vi "Send Hardware Reference.vi"(8 "error in":errorcluster, 11 "Controller in":refnum<class "Controller.lvclass">) -> (0 "error out":errorcluster, 2 "System Hardware Reference":refnum<data-value>, 3 "Controller out":refnum<class "Controller.lvclass">)   [LabVIEW 2016, in "SMI.lvlib" / "Controller.lvclass"]
uses:
  Controller.lvclass
  Controller.lvclass/Controller.ctl
  Accessor Methods/Read System Hardware Reference.vi
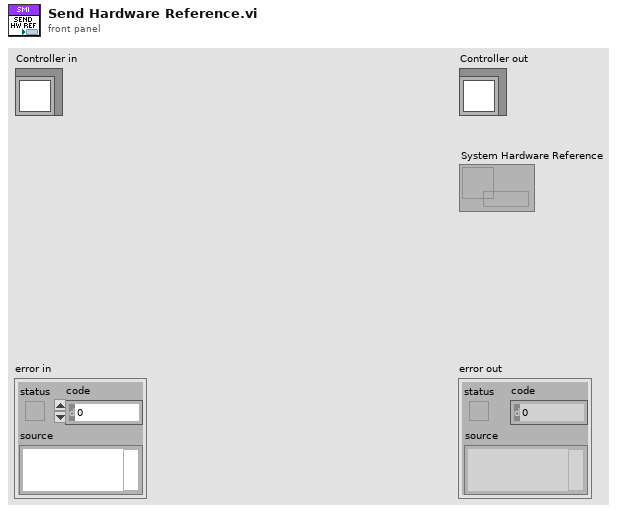
[diagram p1: front panel]
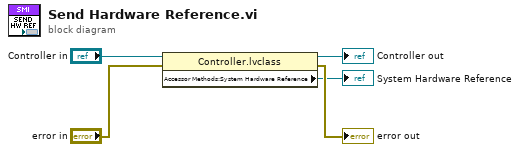
[diagram p0: block diagram]
diagram:
  n1 = property class="Controller.lvclass"(reference="Controller in", error in="error in") -> (reference out=→"Controller out":refnum<class "Controller.lvclass">, error out=→"error out":errorcluster, "Accessor Methods:System Hardware Reference"=→"System Hardware Reference":refnum<data-value>)
